vi "Cut_Out_Short_Subtracks-1.vi"(4 "error IN":errorcluster, 7 "[IN] Subtracks in Row":T1(array[cluster])) -> (0 "error OUT":errorcluster, 1 "[OUT] Indicies of subttracks\nin initial row with them":i32[](array[numeric]), 2 "[OUT] Some tracks are empty":bool, 3 "[OUT Subtracks in Row":T1(array[cluster]))   [LabVIEW 2017]
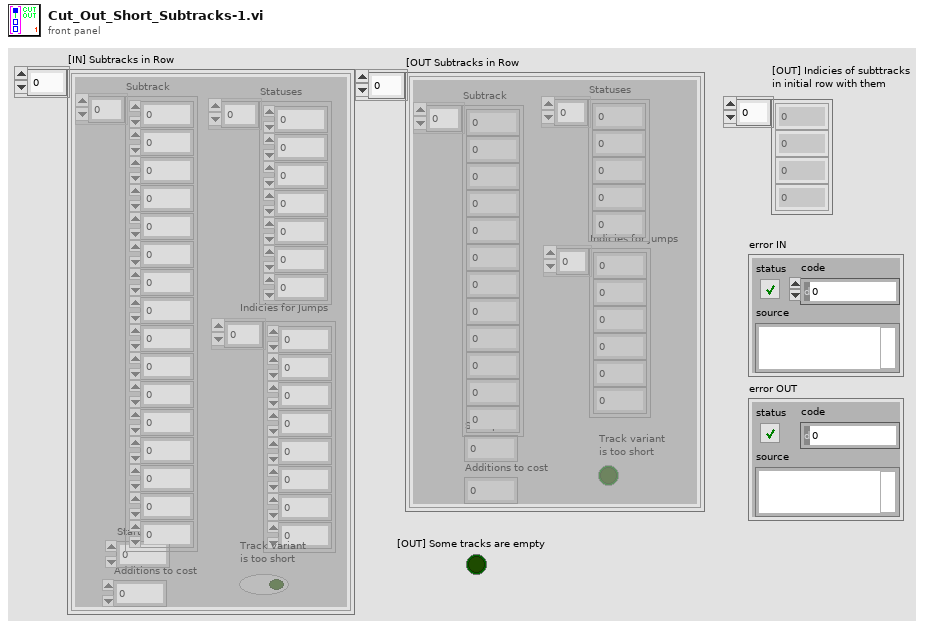
[diagram p1: front panel]
types:
  T1 = cluster{"Subtrack":dbl[], "Statuses":i16[], "Start pos":i32, "Additions to cost":i8, "Track variant \nis too short":bool, "Indicies for Jumps":i32[]}[]
  T2 = cluster{"Subtrack":dbl[], "Statuses":i16[], "Start pos":i32, "Additions to cost":i8, "Track variant \nis too short":bool, "Indicies for Jumps":i32[]}
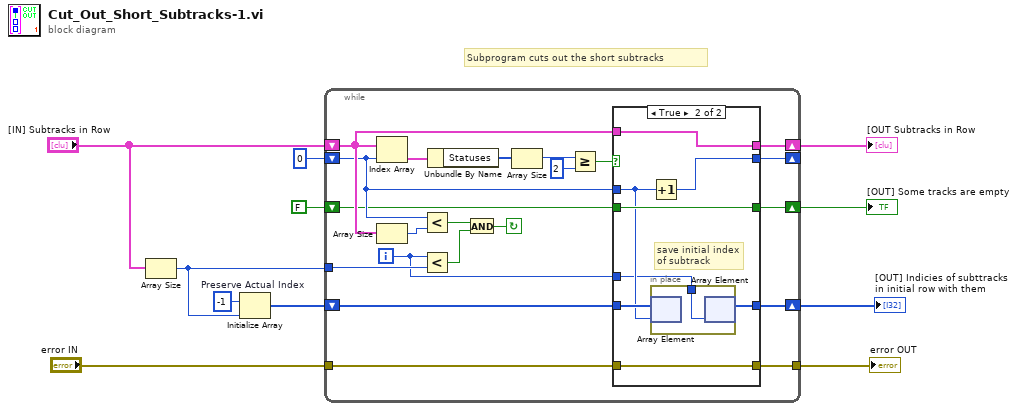
[diagram p0: block diagram]
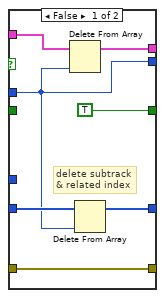
[diagram p2: hidden frame]
diagram:
  # "Subprogram cuts out the short subtracks"
  n1 = Array Size(array="[IN] Subtracks in Row") -> (size(s)=w3:i32)
  n2 = Initialize Array "Preserve Actual Index"(-1 ("element"), w3) -> (w2:i32[])
  n3 = while {
    shift-right: [w27] -> w7
    shift-left: "[IN] Subtracks in Row" -> [w25]
    shift-right: [w26] -> _
    shift-left: 0 -> [w24]
    tunnel: w3 -> [w21]
    tunnel: "error IN" -> [w13]
    tunnel: [w12] -> w8
    shift-right: [w18] -> w5
    shift-left: FALSE -> [w17]
    shift-right: [w15] -> w1
    shift-left: w2 -> [w16]
    i -> [w14]
    stop <- w19 continue-if-true
    n4 = Index Array(array=w25, index=w24) -> (element=w32:T2)
    n5 = Array Size(array=w25) -> (size(s)=w23:i32)
    n6 = Less?(x=w24, y=w23) -> (x < y?=w22:bool)
    n7 = Less?(x=w14, y=w21) -> (x < y?=w20:bool)
    n8 = Unbundle By Name(w32) -> ("Statuses"=w31:i16[])
    n9 = And(x=w22, y=w20) -> (x .and. y?=w19:bool)
    n10 = Array Size(array=w31) -> (size(s)=w30:i32)
    n11 = Greater Or Equal?(x=w30, y=2) -> (x >= y?=w28:bool)
    n12 = case shown="True" w28 {
      tunnel: w25 -> [w39 w47]
      tunnel: [w38 w47] -> w27
      tunnel: w24 -> [w35 w43]
      tunnel: [w35 w46] -> w26
      tunnel: [TRUE w45] -> w18
      tunnel: w17 -> [_ w45]
      tunnel: w16 -> [w36 w44]
      tunnel: [w34 w42] -> w15
      tunnel: w14 -> [_ w41]
      tunnel: w13 -> [w33 w40]
      tunnel: [w33 w40] -> w12
      frame False {
        # "delete subtrack\n& related index"
        n13 = Delete From Array(array=w39, index=w35) -> (array with subset deleted=w38:T1)  [unwired: 1 in, 1 out]
        n14 = Delete From Array(array=w36, index=w35) -> (array with subset deleted=w34:i32[])  [unwired: 1 in, 1 out]
      }
      frame True {
        # "save initial index\nof subtrack"
        n15 = Increment(x=w43) -> (x+1=w46:i32)
        n16 = in-place {
          in-place-border: w41 -> [w48]
          n17 = in-place-array #1(w44, w43) -> ()  [unwired: 1 out]
          n18 = in-place-array #1(w48) -> (w42:i32[])  [unwired: 1 out]
        }
      }
    }
  }
  "error OUT" <- w8
  "[OUT Subtracks in Row" <- w7
  "[OUT] Some tracks are empty" <- w5
  "[OUT] Indicies of subttracks\nin initial row with them" <- w1
